vi "Read.vi"(8 "error in (no error)":errorcluster, 10 "delay before read (100ms)":u32=10, 11 "Serial in":refnum<class "Serial.lvclass">) -> (0 "error out":errorcluster, 3 "Serial out":refnum<class "Serial.lvclass">)   [LabVIEW 2019, in "Serial.lvlib" / "Serial.lvclass"]
uses:
  Serial.lvclass
  C:/Program Files (x86)/National Instruments/LabVIEW 2019/vi.lib/ActorFramework/Actor/Actor.lvclass
  Serial.lvclass/Serial.ctl
  <vilib>/ActorFramework/Actor/Actor.lvclass/Actor.ctl
  Serial Messages/Response Msg/Response Msg.lvclass/Response Msg.ctl
  <vilib>/ActorFramework/Message Enqueuer/Message Enqueuer.lvclass/Message Enqueuer.ctl
  <vilib>/ActorFramework/Message Enqueuer/Enqueue.vi
  Serial Messages/Response Msg/Response Msg.lvclass
  C:/Program Files (x86)/National Instruments/LabVIEW 2019/vi.lib/ActorFramework/Message/Message.lvclass
  <vilib>/ActorFramework/Message Priority Queue/Priority Enqueue.vi
  <vilib>/ActorFramework/Actor/Actor.lvclass
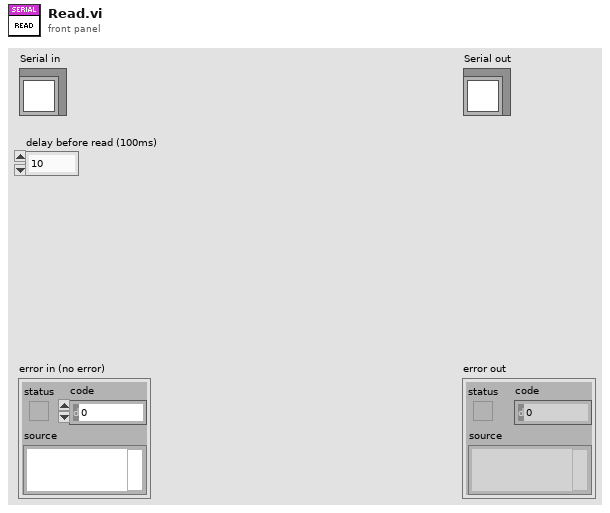
[diagram p1: front panel]
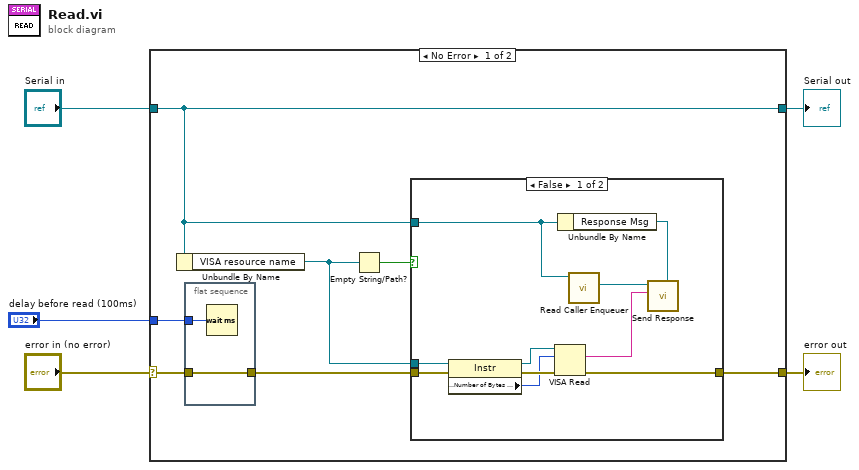
[diagram p0: block diagram]
diagram:
  n1 = case shown="No Error" "error in (no error)" {
    selector: "error in (no error)" -> [w11 w27]
    tunnel: [w10 w27] -> w4
    tunnel: [w7 w26] -> w2
    tunnel: "Serial in" -> [w7 w26]
    tunnel: "delay before read (100ms)" -> [w9 _]
    frame No Error {
      n2 = Unbundle By Name(w7) -> ("VISA resource name"=w8:refnum<visa-resource-name>)
      n3 = flat-sequence {
        tunnel: w11 -> [w25]
        tunnel: [w25] -> w12
        tunnel: w9 -> [w24]
        frame #0 {
          n4 = Wait (ms)(milliseconds to wait=w24) -> ()  [unwired: 1 out]
        }
      }
      n5 = Empty String/Path?(string/path=w8) -> (empty?=w6:bool)
      n6 = case shown="False" w6 {
        tunnel: w12 -> [w22 w23]
        tunnel: [w21 w23] -> w10
        tunnel: w8 -> [w17 _]
        tunnel: w7 -> [w13 _]
        frame False {
          n7 = property class="Instr"(reference=w17, error in=w22) -> (reference out=w15:refnum<visa-resource-name>, error out=w16:errorcluster, "Serial Settings:Number of Bytes at Serial Port"=w14:u32)
          n8 = VISA Read(VISA resource name=w15, byte count=w14, error in (no error)=w16) -> (read buffer=w18:string, error out=w21:errorcluster)  [unwired: 2 out]
          n9 = Unbundle By Name(w13) -> ("Response Msg"=w20:refnum<class "Response Msg.lvclass">)
          n10 = call <vilib>:"Read Caller Enqueuer.vi"("Actor"=w13) -> ("Caller Enqueuer"=w19:refnum<class "Message Enqueuer.lvclass">)  [unwired: 10 in]
          n11 = call "Send Response.vi"("Message Type"=w20, "Response"=w18, "Message Enqueuer"=w19) -> ()  [unwired: 7 in, 2 out]
        }
        frame True {
        }
      }
    }
    frame Error {
    }
  }
  "error out" <- w4
  "Serial out" <- w2
